vi "Test Inverse F CDF.vi"() -> ()   [LabVIEW 2021, in "Math.lvlib"]
uses:
  Arrays/Linear Ramp End Options.ctl
  b0ce6316-0586-4496-b7d9-1a99ffc9eed6.vi
  <vilib>/gmath/statdist.llb/F Inverse CDF.vi
  Math/Math.lvlib
  <vilib>/gmath/NI_Gmath.lvlib
  Arrays/Arrays.lvlib
panel:
  in  "CL":dbl=0.05 format="%#_13g"
  out "XY Graph":cluster{"Ramp":dbl[], dbl[]}[](graph)
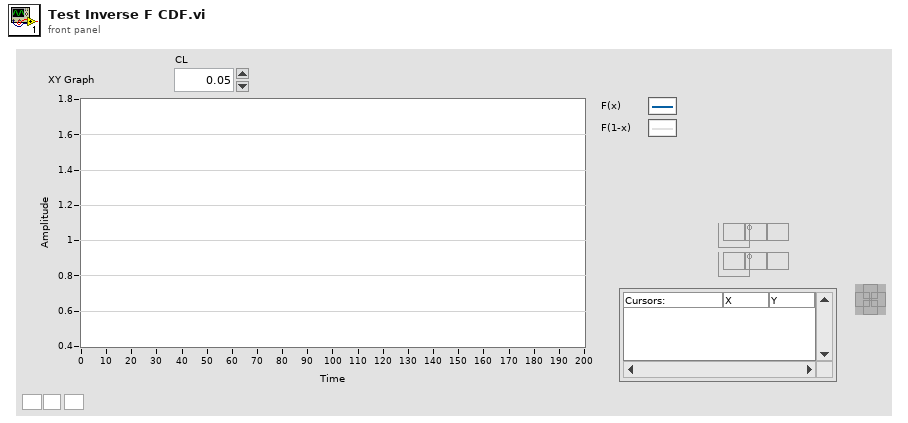
[diagram p1: front panel]
types:
  T1 = typedef "Arrays.lvlib/Linear Ramp End Options.ctl" = enum16{"Include Min/Exclude Max", "Exclude Min/Include Max", "Include Both Ends", "Exclude Both Ends"}
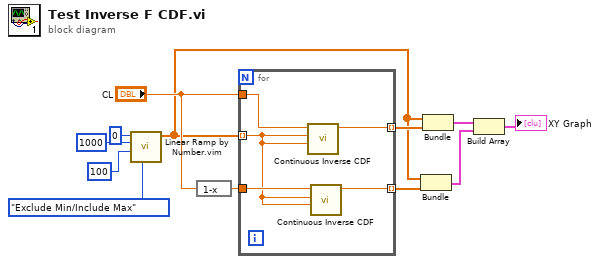
[diagram p0: block diagram]
diagram:
  n1 = call "Linear Ramp by Number.vim"("Options"=Linear_Ramp_End_Options."Exclude Min/Include Max", "# Steps (1)"=100, "End (1)"=1000, "Start (0)"=0) -> ("Ramp"=w2:dbl[])  [unwired: 5 in, 2 out]
  n2 = expression code="1-x"("CL") -> (w4:dbl)
  n3 = for {
    tunnel: w2 -> [w14] mode=indexing
    tunnel: [w17] -> w8 mode=indexing
    tunnel: "CL" -> [w16]
    tunnel: w4 -> [w15]
    tunnel: [w13] -> w3 mode=indexing
    n4 = call-poly <vilib>:"Continuous Inverse CDF.vi"("k2"=w14, "k1"=w14, "cdf(x)"=w16) -> ("x"=w17:dbl)  [unwired: 7 in, 1 out]
    n5 = call-poly <vilib>:"Continuous Inverse CDF.vi"("k2"=w14, "k1"=w14, "cdf(x)"=w15) -> ("x"=w13:dbl)  [unwired: 7 in, 1 out]
  }
  n6 = Bundle("Ramp"=w2, w3) -> (w1:cluster{"Ramp":dbl[], dbl[]})  [unwired: 1 in]
  n7 = Bundle("Ramp"=w2, w8) -> (w7:cluster{"Ramp":dbl[], dbl[]})  [unwired: 1 in]
  n8 = Build Array(w7, w1) -> (→"XY Graph":cluster{"Ramp":dbl[], dbl[]}[])
